vi "Coinc to save format.vi"(1 "Coincidences":T1) -> (0 "Array":T3(array[cluster]))   [LabVIEW 2016]
uses:
  Typedefs/CoincidencesToSave.ctl
  Typedefs/CoincidenceWithGPSformat.ctl
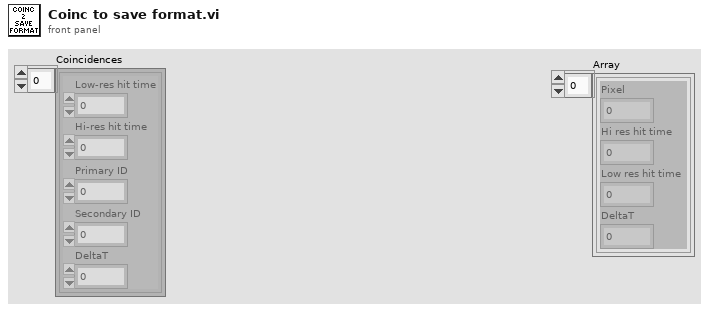
[diagram p1: front panel]
types:
  T1 = typedef "CoincidencesToSave.ctl" = T2[]
  T2 = typedef "CoincidenceWithGPSformat.ctl" = cluster{"Low-res hit time":u32, "Hi-res hit time":u32, "Secondary ID":i8, "DeltaT":i32, "Primary ID":i8}
  T3 = cluster{"Pixel":i8, "Hi res hit time":u32, "Low res hit time":u32, "DeltaT":i16}[]
  T4 = cluster{"Pixel":i8, "Hires hit time":u32, "Lowres hit time":u32, "DeltaT":i16}
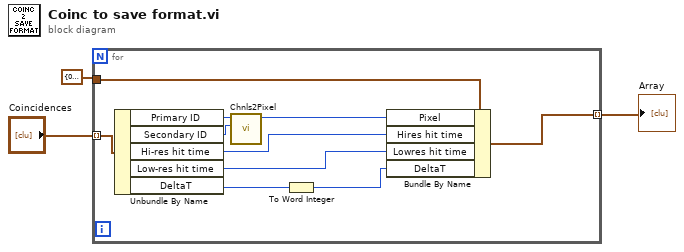
[diagram p0: block diagram]
diagram:
  n1 = for {
    tunnel: "Coincidences" -> [w13] mode=indexing
    tunnel: [w8] -> w3 mode=indexing
    tunnel: T4 {"Pixel"=0, "Hires hit time"=0, "Lowres hit time"=0, "DeltaT"=0} -> [w7]
    n2 = Unbundle By Name(w13) -> ("Primary ID"=w12:i8, "Secondary ID"=w11:i8, "Hi-res hit time"=w9:u32, "Low-res hit time"=w6:u32, "DeltaT"=w5:i32)
    n3 = call "Chnls2Pixel.vi"("Secondary"=w11, "Primary"=w12) -> ("Pixel ID"=w10:i8)  [unwired: 9 in]
    n4 = To Word Integer(number=w5) -> (16bit integer=w4:i16)
    n5 = Bundle By Name(cluster=w7, "Pixel"=w10, "Hires hit time"=w9, "Lowres hit time"=w6, "DeltaT"=w4) -> (w8:T4)
  }
  "Array" <- w3
